vi "Rotate Vector.vi"(10 "Angle [rad]":dbl, 11 "Vector":dbl[](array[numeric])) -> (3 "Rotated vector":dbl[](array[numeric]))   [LabVIEW 2020, in "Spinner.lvlib"]
uses:
  Spinner.lvlib
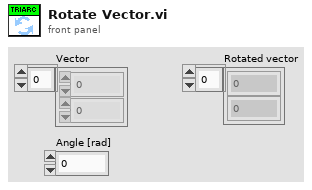
[diagram p1: front panel]
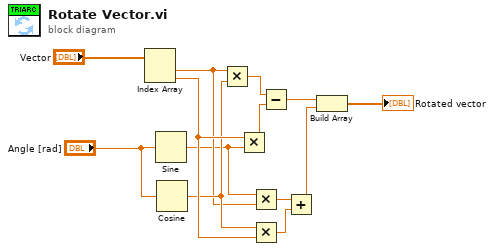
[diagram p0: block diagram]
diagram:
  n1 = Index Array(array="Vector") -> (element #1=w7:dbl, element #2=w9:dbl)  [unwired: 2 in]
  n2 = Sine(x="Angle [rad]") -> (sin(x)=w6:dbl)
  n3 = Cosine(x="Angle [rad]") -> (cos(x)=w8:dbl)
  n4 = Multiply(x=w7, y=w8) -> (x*y=w3:dbl)
  n5 = Multiply(x=w9, y=w6) -> (x*y=w4:dbl)
  n6 = Multiply(x=w6, y=w7) -> (x*y=w10:dbl)
  n7 = Multiply(x=w8, y=w9) -> (x*y=w11:dbl)
  n8 = Subtract(x=w3, y=w4) -> (x-y=w5:dbl)
  n9 = Add(x=w10, y=w11) -> (x+y=w12:dbl)
  n10 = Build Array(w5, w12) -> (→"Rotated vector":dbl[])
